vi "Write System Data.vi"(8 "Error In":errorcluster, 9 "AFV-P System Data":T1 {"Freq Lo Limit" format="%#.1f Hz"; "Freq Hi Limit" format="%#.1f Hz"; "Volt Lo Limit" format="%.1f V"; "Volt Hi Limit" format="%.1f V"; "DC Volt Lo Limit" format="%.1f V"; "DC Volt Hi Limit" format="%.1f V"}, 10 "Modbus ID":string, 11 "VISA resource name":refnum<visa-resource-name>) -> (0 "Error Out":errorcluster, 3 "VISA resource name out":refnum<visa-resource-name>)   [LabVIEW 2013]
panel:
  # "."
  # "."
  # "."
  # "."
  # "."
  # "."
  # "."
  # "."
  # "."
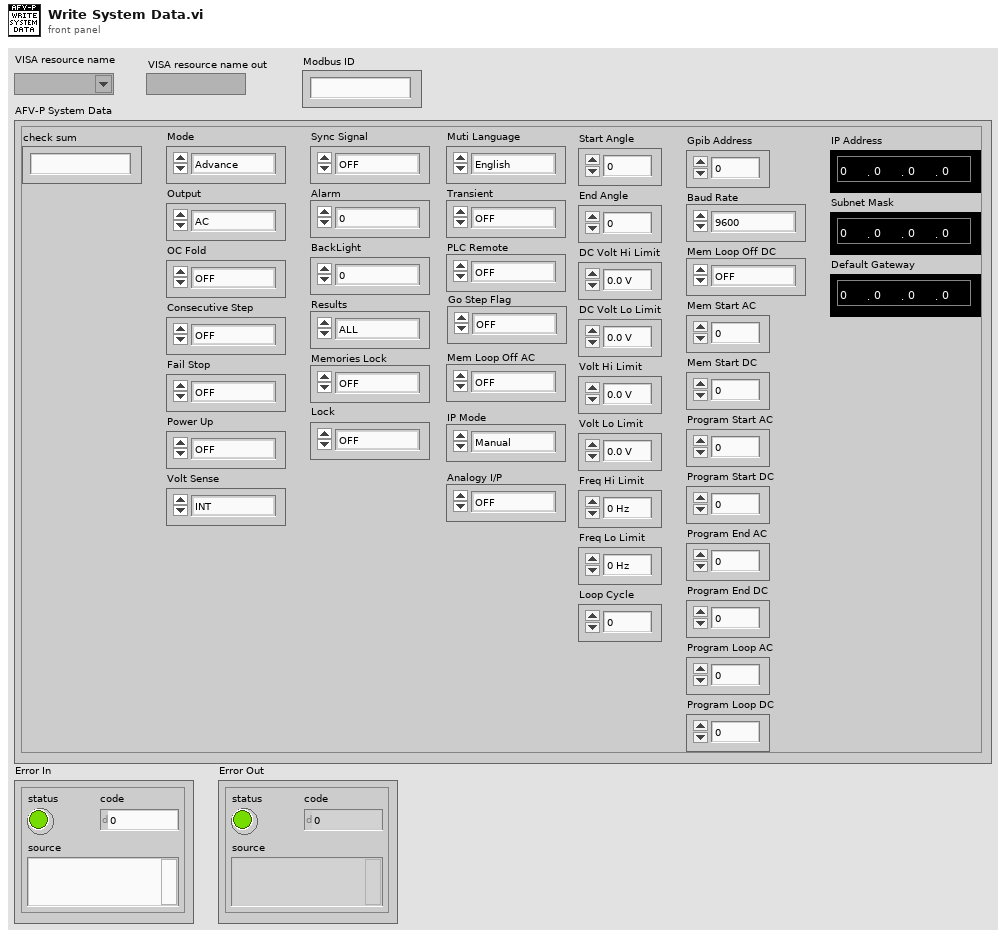
[diagram p1: front panel]
types:
  T1 = cluster{"check sum":string, "Mode":enum16{"Advance", "Basic"}, "Output":enum16{"AC", "DC"}, "OC Fold":enum16{"OFF", "ON"}, "Consecutive Step":enum16{"OFF", "ON"}, "Fail Stop":enum16{"OFF", "ON"}, "Power Up":enum16{"OFF", "ON", "LAST"}, "Volt Sense":enum16{"INT", "EXT"}, "Sync Signal":enum16{"OFF", "ON", "EVENT"}, "Alarm":enum16{"0", "1", "2", "3", "4", "5", "6", "7", "8", "9"}, "BackLight":enum16{"0", "1", "2", "3", "4", "5", "6", "7", "8", "9"}, "Results":enum16{"ALL", "P/F", "LAST"}, "Memories Lock":enum16{"OFF", "ON"}, "Lock":enum16{"OFF", "ON"}, "Muti Language":enum16{"English", "繁體中文", "簡體中文", "日文"}, "Transient":enum16{"OFF", "ON"}, "PLC Remote":enum16{"OFF", "ON"}, "Go Step Flag":enum16{"OFF", "ON"}, "Mem Loop Off AC":enum16{"OFF", "ON"}, "IP Mode":enum16{"Manual", "Auto"}, "Analogy I/P":enum16{"OFF", "ON"}, "Start Angle":u16, "End Angle":u16, "DC Volt Hi Limit":dbl, "DC Volt Lo Limit":dbl, "Volt Hi Limit":dbl, "Volt Lo Limit":dbl, "Freq Hi Limit":dbl, "Freq Lo Limit":dbl, "Loop Cycle":u16, "Gpib Address":u8, "Baud Rate":enum16{"9600", "19200", "38400", "57600", "115200"}, "Mem Loop Off DC":enum16{"OFF", "ON"}, "Mem Start AC":u8, "Mem Start DC":u8, "Program Start AC":u16, "Program Start DC":u16, "Program End AC":u16, "Program End DC":u16, "Program Loop AC":u16, "Program Loop DC":u16, "IP Address":cluster{"IP 0":u8, "IP 1":u8, "IP 2":u8, "IP 3":u8}, "Subnet Mask":cluster{"IP 0":u8, "IP 1":u8, "IP 2":u8, "IP 3":u8}, "Default Gateway":cluster{"IP 0":u8, "IP 1":u8, "IP 2":u8, "IP 3":u8}}
  T2 = cluster{"ID":string, "Function Code":string, "Length (High)":string, "Length (Low)":string, "Start Address (High)":string, "Start Address (Middle High)":string, "Start Address (Middle Low)":string, "Start Address (Low)":string, "Data":string}
  T3 = enum16{"0", "1", "2", "3", "4", "5", "6", "7", "8", "9"}
  T4 = enum16{"9600", "19200", "38400", "57600", "115200"}
  T5 = cluster{"Length (High)":string, "Length (Low)":string, "Start Address (High)":string, "Start Address (Middle High)":string, "Start Address (Middle Low)":string, "Start Address (Low)":string}
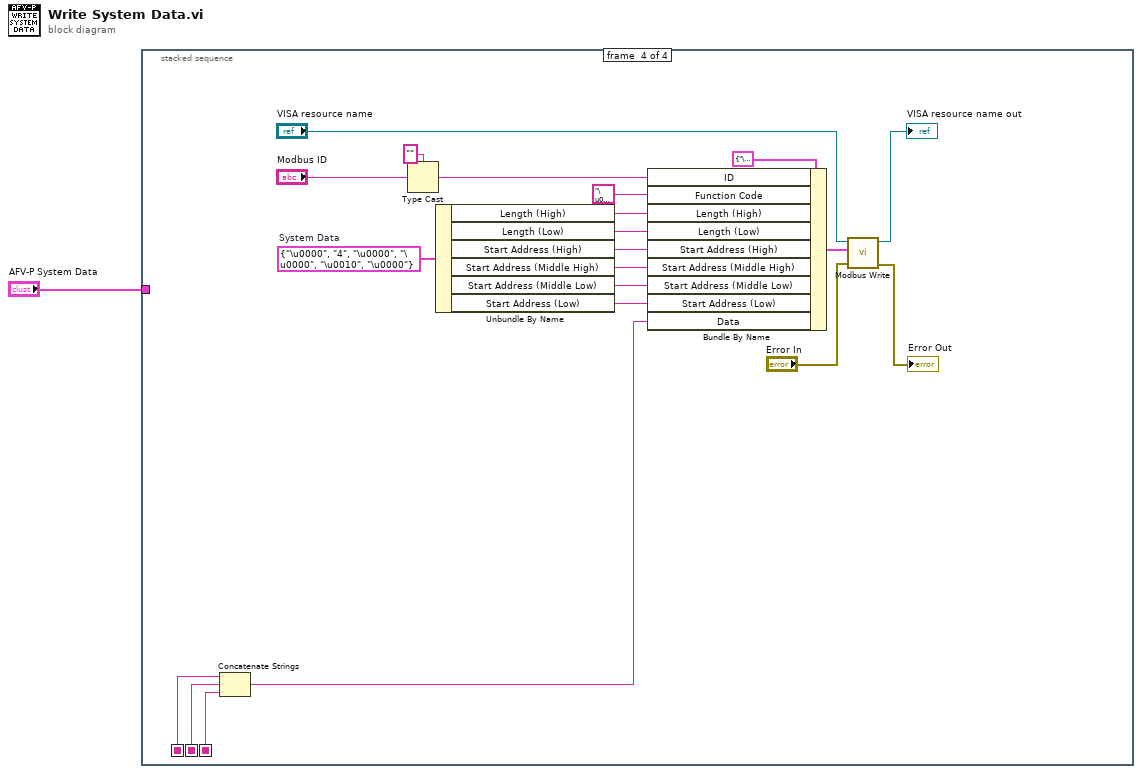
[diagram p0: block diagram]
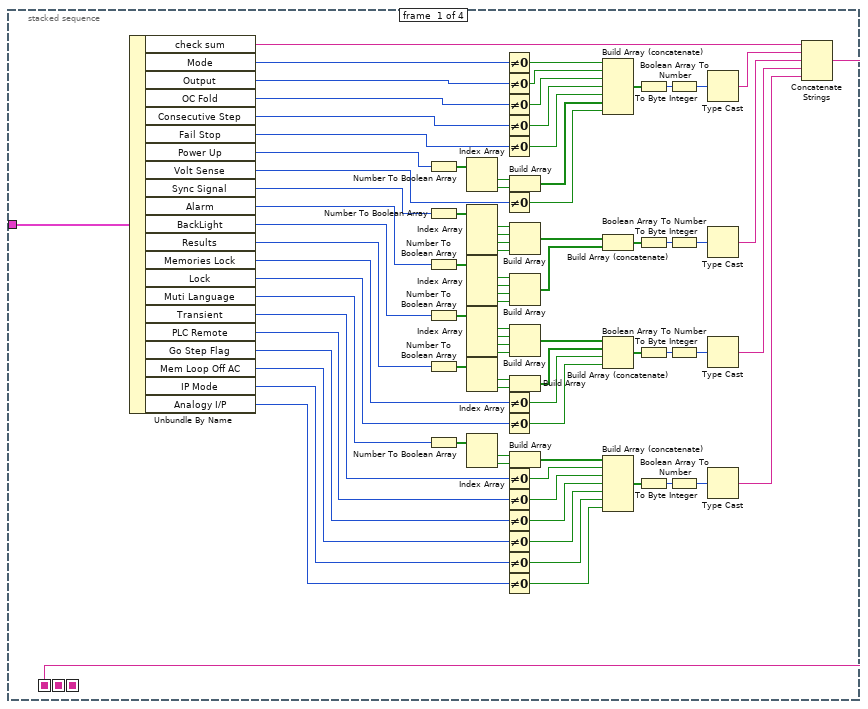
[diagram p2: hidden frame]
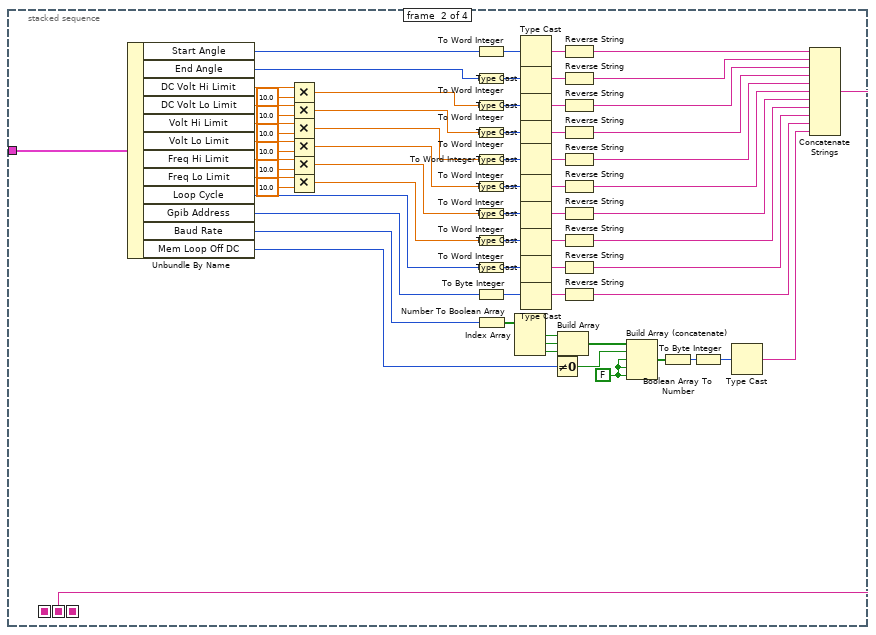
[diagram p3: hidden frame]
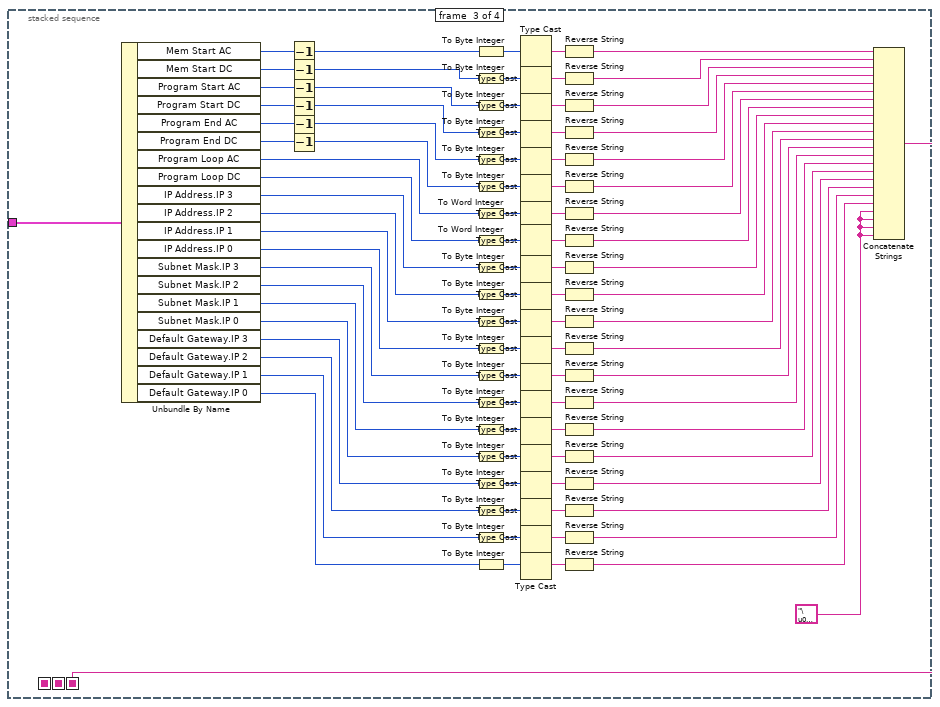
[diagram p4: hidden frame]
diagram:
  n1 = stacked-sequence {
    seq-local: [w11 _ _ _] -> [_ _ _ w261]
    seq-local: [_ w151 _ _] -> [_ _ _ w260]
    seq-local: [_ _ w217 _] -> [_ _ _ w259]
    tunnel: "AFV-P System Data" -> [w2 w85 w152 _]
    frame #0 {
      n2 = Unbundle By Name(w2) -> ("check sum"=w84:string, "Mode"=w83:enum16{"Advance", "Basic"}, "Output"=w82:enum16{"AC", "DC"}, "OC Fold"=w81:enum16{"OFF", "ON"}, "Consecutive Step"=w80:enum16{"OFF", "ON"}, "Fail Stop"=w79:enum16{"OFF", "ON"}, "Power Up"=w75:enum16{"OFF", "ON", "LAST"}, "Volt Sense"=w65:enum16{"INT", "EXT"}, "Sync Signal"=w59:enum16{"OFF", "ON", "EVENT"}, "Alarm"=w51:T3, "BackLight"=w39:T3, "Results"=w35:enum16{"ALL", "P/F", "LAST"}, "Memories Lock"=w34:enum16{"OFF", "ON"}, "Lock"=w33:enum16{"OFF", "ON"}, "Muti Language"=w21:enum16{"English", "繁體中文", "簡體中文", "日文"}, "Transient"=w20:enum16{"OFF", "ON"}, "PLC Remote"=w19:enum16{"OFF", "ON"}, "Go Step Flag"=w9:enum16{"OFF", "ON"}, "Mem Loop Off AC"=w8:enum16{"OFF", "ON"}, "IP Mode"=w7:enum16{"Manual", "Auto"}, "Analogy I/P"=w6:enum16{"OFF", "ON"})
      n3 = Number To Boolean Array(number=w75) -> (Boolean array=w78:bool[])
      n4 = Number To Boolean Array(number=w59) -> (Boolean array=w60:bool[])
      n5 = Number To Boolean Array(number=w51) -> (Boolean array=w54:bool[])
      n6 = Number To Boolean Array(number=w39) -> (Boolean array=w42:bool[])
      n7 = Number To Boolean Array(number=w35) -> (Boolean array=w36:bool[])
      n8 = Number To Boolean Array(number=w21) -> (Boolean array=w24:bool[])
      n9 = Index Array(array=w78) -> (element #1=w77:bool, element #2=w76:bool)  [unwired: 2 in]
      n10 = Index Array(array=w60) -> (element #1=w61:bool, element #2=w62:bool, element #3=w58:bool, element #4=w57:bool)  [unwired: 4 in]
      n11 = Index Array(array=w54) -> (element #1=w53:bool, element #2=w52:bool, element #3=w55:bool, element #4=w56:bool)  [unwired: 4 in]
      n12 = Index Array(array=w42) -> (element #1=w43:bool, element #2=w44:bool, element #3=w41:bool, element #4=w40:bool)  [unwired: 4 in]
      n13 = Index Array(array=w36) -> (element #1=w37:bool, element #2=w38:bool)  [unwired: 2 in]
      n14 = Index Array(array=w24) -> (element #1=w23:bool, element #2=w22:bool)  [unwired: 2 in]
      n15 = Not Equal To 0?(x=w83) -> (x != 0?=w71:bool)
      n16 = Not Equal To 0?(x=w82) -> (x != 0?=w70:bool)
      n17 = Not Equal To 0?(x=w81) -> (x != 0?=w69:bool)
      n18 = Not Equal To 0?(x=w80) -> (x != 0?=w68:bool)
      n19 = Not Equal To 0?(x=w79) -> (x != 0?=w67:bool)
      n20 = Not Equal To 0?(x=w65) -> (x != 0?=w64:bool)
      n21 = Not Equal To 0?(x=w34) -> (x != 0?=w30:bool)
      n22 = Not Equal To 0?(x=w33) -> (x != 0?=w29:bool)
      n23 = Not Equal To 0?(x=w20) -> (x != 0?=w14:bool)
      n24 = Not Equal To 0?(x=w19) -> (x != 0?=w13:bool)
      n25 = Not Equal To 0?(x=w9) -> (x != 0?=w10:bool)
      n26 = Not Equal To 0?(x=w8) -> (x != 0?=w5:bool)
      n27 = Not Equal To 0?(x=w7) -> (x != 0?=w4:bool)
      n28 = Not Equal To 0?(x=w6) -> (x != 0?=w3:bool)
      n29 = Build Array(w77, w76) -> (w66:bool[])
      n30 = Build Array(w61, w62, w58, w57) -> (w47:bool[])
      n31 = Build Array(w53, w52, w55, w56) -> (w46:bool[])
      n32 = Build Array(w43, w44, w41, w40) -> (w32:bool[])
      n33 = Build Array(w37, w38) -> (w31:bool[])
      n34 = Build Array(w23, w22) -> (w15:bool[])
      n35 = Build Array (concatenate)(w71, w70, w69, w68, w67, w66, w64) -> (w74:bool[])
      n36 = Build Array (concatenate)(w47, w46) -> (w48:bool[])
      n37 = Build Array (concatenate)(w32, w31, w30, w29) -> (w26:bool[])
      n38 = Build Array (concatenate)(w15, w14, w13, w10, w5, w4, w3) -> (w18:bool[])
      n39 = Boolean Array To Number(Boolean array=w74) -> (number=w73:u32)
      n40 = Boolean Array To Number(Boolean array=w48) -> (number=w49:u32)
      n41 = Boolean Array To Number(Boolean array=w26) -> (number=w28:u32)
      n42 = Boolean Array To Number(Boolean array=w18) -> (number=w16:u32)
      n43 = To Byte Integer(number=w73) -> (8bit integer=w72:i8)
      n44 = To Byte Integer(number=w49) -> (8bit integer=w50:i8)
      n45 = To Byte Integer(number=w28) -> (8bit integer=w27:i8)
      n46 = To Byte Integer(number=w16) -> (8bit integer=w17:i8)
      n47 = Type Cast(x=w72) -> (*(type *) &x=w63:string)  [unwired: 1 in]
      n48 = Type Cast(x=w50) -> (*(type *) &x=w45:string)  [unwired: 1 in]
      n49 = Type Cast(x=w27) -> (*(type *) &x=w25:string)  [unwired: 1 in]
      n50 = Type Cast(x=w17) -> (*(type *) &x=w12:string)  [unwired: 1 in]
      n51 = Concatenate Strings(w84, w63, w45, w25, w12) -> (w11:string)
    }
    frame #1 {
      w98 = FALSE
      n52 = Unbundle By Name(w85) -> ("Start Angle"=w148:u16, "End Angle"=w144:u16, "DC Volt Hi Limit"=w102:dbl, "DC Volt Lo Limit"=w100:dbl, "Volt Hi Limit"=w111:dbl, "Volt Lo Limit"=w119:dbl, "Freq Hi Limit"=w116:dbl, "Freq Lo Limit"=w114:dbl, "Loop Cycle"=w128:u16, "Gpib Address"=w123:u8, "Baud Rate"=w88:T4, "Mem Loop Off DC"=w87:enum16{"OFF", "ON"})
      n53 = Multiply(x=w102, y=10.0) -> (x*y=w101:dbl)
      n54 = Multiply(x=w100, y=10.0) -> (x*y=w99:dbl)
      n55 = Multiply(x=w111, y=10.0) -> (x*y=w121:dbl)
      n56 = Multiply(x=w119, y=10.0) -> (x*y=w118:dbl)
      n57 = Multiply(x=w116, y=10.0) -> (x*y=w115:dbl)
      n58 = Multiply(x=w114, y=10.0) -> (x*y=w112:dbl)
      n59 = To Word Integer(number=w148) -> (16bit integer=w149:i16)
      n60 = To Word Integer(number=w144) -> (16bit integer=w146:i16)
      n61 = To Word Integer(number=w101) -> (16bit integer=w108:i16)
      n62 = To Word Integer(number=w99) -> (16bit integer=w109:i16)
      n63 = To Word Integer(number=w121) -> (16bit integer=w141:i16)
      n64 = To Word Integer(number=w118) -> (16bit integer=w139:i16)
      n65 = To Word Integer(number=w115) -> (16bit integer=w135:i16)
      n66 = To Word Integer(number=w112) -> (16bit integer=w133:i16)
      n67 = To Word Integer(number=w128) -> (16bit integer=w129:i16)
      n68 = To Byte Integer(number=w123) -> (8bit integer=w126:i8)
      n69 = Number To Boolean Array(number=w88) -> (Boolean array=w95:bool[])
      n70 = Index Array(array=w95) -> (element #1=w96:bool, element #2=w97:bool, element #3=w94:bool)  [unwired: 3 in]
      n71 = Type Cast(x=w149) -> (*(type *) &x=w150:string)  [unwired: 1 in]
      n72 = Type Cast(x=w146) -> (*(type *) &x=w145:string)  [unwired: 1 in]
      n73 = Type Cast(x=w108) -> (*(type *) &x=w107:string)  [unwired: 1 in]
      n74 = Type Cast(x=w109) -> (*(type *) &x=w110:string)  [unwired: 1 in]
      n75 = Type Cast(x=w141) -> (*(type *) &x=w142:string)  [unwired: 1 in]
      n76 = Type Cast(x=w139) -> (*(type *) &x=w138:string)  [unwired: 1 in]
      n77 = Type Cast(x=w135) -> (*(type *) &x=w136:string)  [unwired: 1 in]
      n78 = Type Cast(x=w133) -> (*(type *) &x=w132:string)  [unwired: 1 in]
      n79 = Type Cast(x=w129) -> (*(type *) &x=w130:string)  [unwired: 1 in]
      n80 = Type Cast(x=w126) -> (*(type *) &x=w125:string)  [unwired: 1 in]
      n81 = Not Equal To 0?(x=w87) -> (x != 0?=w86:bool)
      n82 = Build Array(w96, w97, w94) -> (w93:bool[])
      n83 = Reverse String(1:w150) -> (0:w147:string)
      n84 = Reverse String(1:w145) -> (0:w143:string)
      n85 = Reverse String(1:w107) -> (0:w106:string)
      n86 = Reverse String(1:w110) -> (0:w105:string)
      n87 = Reverse String(1:w142) -> (0:w140:string)
      n88 = Reverse String(1:w138) -> (0:w137:string)
      n89 = Reverse String(1:w136) -> (0:w134:string)
      n90 = Reverse String(1:w132) -> (0:w131:string)
      n91 = Reverse String(1:w130) -> (0:w127:string)
      n92 = Reverse String(1:w125) -> (0:w124:string)
      n93 = Build Array (concatenate)(w93, w86, w98, w98, w98) -> (w90:bool[])
      n94 = Boolean Array To Number(Boolean array=w90) -> (number=w92:u32)
      n95 = To Byte Integer(number=w92) -> (8bit integer=w91:i8)
      n96 = Type Cast(x=w91) -> (*(type *) &x=w89:string)  [unwired: 1 in]
      n97 = Concatenate Strings(w147, w143, w106, w105, w140, w137, w134, w131, w127, w124, w89) -> (w151:string)
    }
    frame #2 {
      w176 = "\u0000" ("string")
      n98 = Unbundle By Name(w152) -> ("Mem Start AC"=w238:u8, "Mem Start DC"=w232:u8, "Program Start AC"=w231:u16, "Program Start DC"=w159:u16, "Program End AC"=w158:u16, "Program End DC"=w157:u16, "Program Loop AC"=w156:u16, "Program Loop DC"=w160:u16, "IP Address.IP 3"=w216:u8, "IP Address.IP 2"=w215:u8, "IP Address.IP 1"=w214:u8, "IP Address.IP 0"=w194:u8, "Subnet Mask.IP 3"=w193:u8, "Subnet Mask.IP 2"=w192:u8, "Subnet Mask.IP 1"=w191:u8, "Subnet Mask.IP 0"=w190:u8, "Default Gateway.IP 3"=w189:u8, "Default Gateway.IP 2"=w188:u8, "Default Gateway.IP 1"=w187:u8, "Default Gateway.IP 0"=w186:u8)
      n99 = Decrement(x=w238) -> (x-1=w167:u8)
      n100 = Decrement(x=w232) -> (x-1=w219:u8)
      n101 = Decrement(x=w231) -> (x-1=w218:u16)
      n102 = Decrement(x=w159) -> (x-1=w155:u16)
      n103 = Decrement(x=w158) -> (x-1=w154:u16)
      n104 = Decrement(x=w157) -> (x-1=w153:u16)
      n105 = To Byte Integer(number=w167) -> (8bit integer=w240:i8)
      n106 = To Byte Integer(number=w219) -> (8bit integer=w233:i8)
      n107 = To Byte Integer(number=w218) -> (8bit integer=w236:i8)
      n108 = To Byte Integer(number=w155) -> (8bit integer=w170:i8)
      n109 = To Byte Integer(number=w154) -> (8bit integer=w175:i8)
      n110 = To Byte Integer(number=w153) -> (8bit integer=w172:i8)
      n111 = To Word Integer(number=w156) -> (16bit integer=w168:i16)
      n112 = To Word Integer(number=w160) -> (16bit integer=w230:i16)
      n113 = To Byte Integer(number=w216) -> (8bit integer=w227:i8)
      n114 = To Byte Integer(number=w215) -> (8bit integer=w224:i8)
      n115 = To Byte Integer(number=w214) -> (8bit integer=w213:i8)
      n116 = To Byte Integer(number=w194) -> (8bit integer=w208:i8)
      n117 = To Byte Integer(number=w193) -> (8bit integer=w211:i8)
      n118 = To Byte Integer(number=w192) -> (8bit integer=w212:i8)
      n119 = To Byte Integer(number=w191) -> (8bit integer=w196:i8)
      n120 = To Byte Integer(number=w190) -> (8bit integer=w199:i8)
      n121 = To Byte Integer(number=w189) -> (8bit integer=w200:i8)
      n122 = To Byte Integer(number=w188) -> (8bit integer=w205:i8)
      n123 = To Byte Integer(number=w187) -> (8bit integer=w202:i8)
      n124 = To Byte Integer(number=w186) -> (8bit integer=w201:i8)
      n125 = Type Cast(x=w240) -> (*(type *) &x=w239:string)  [unwired: 1 in]
      n126 = Type Cast(x=w233) -> (*(type *) &x=w234:string)  [unwired: 1 in]
      n127 = Type Cast(x=w236) -> (*(type *) &x=w235:string)  [unwired: 1 in]
      n128 = Type Cast(x=w170) -> (*(type *) &x=w171:string)  [unwired: 1 in]
      n129 = Type Cast(x=w175) -> (*(type *) &x=w174:string)  [unwired: 1 in]
      n130 = Type Cast(x=w172) -> (*(type *) &x=w173:string)  [unwired: 1 in]
      n131 = Type Cast(x=w168) -> (*(type *) &x=w169:string)  [unwired: 1 in]
      n132 = Type Cast(x=w230) -> (*(type *) &x=w229:string)  [unwired: 1 in]
      n133 = Type Cast(x=w227) -> (*(type *) &x=w226:string)  [unwired: 1 in]
      n134 = Type Cast(x=w224) -> (*(type *) &x=w225:string)  [unwired: 1 in]
      n135 = Type Cast(x=w213) -> (*(type *) &x=w228:string)  [unwired: 1 in]
      n136 = Type Cast(x=w208) -> (*(type *) &x=w209:string)  [unwired: 1 in]
      n137 = Type Cast(x=w211) -> (*(type *) &x=w210:string)  [unwired: 1 in]
      n138 = Type Cast(x=w212) -> (*(type *) &x=w207:string)  [unwired: 1 in]
      n139 = Type Cast(x=w196) -> (*(type *) &x=w197:string)  [unwired: 1 in]
      n140 = Type Cast(x=w199) -> (*(type *) &x=w198:string)  [unwired: 1 in]
      n141 = Type Cast(x=w200) -> (*(type *) &x=w195:string)  [unwired: 1 in]
      n142 = Type Cast(x=w205) -> (*(type *) &x=w204:string)  [unwired: 1 in]
      n143 = Type Cast(x=w202) -> (*(type *) &x=w203:string)  [unwired: 1 in]
      n144 = Type Cast(x=w201) -> (*(type *) &x=w206:string)  [unwired: 1 in]
      n145 = Reverse String(1:w239) -> (0:w237:string)
      n146 = Reverse String(1:w234) -> (0:w166:string)
      n147 = Reverse String(1:w235) -> (0:w165:string)
      n148 = Reverse String(1:w171) -> (0:w164:string)
      n149 = Reverse String(1:w174) -> (0:w163:string)
      n150 = Reverse String(1:w173) -> (0:w162:string)
      n151 = Reverse String(1:w169) -> (0:w161:string)
      n152 = Reverse String(1:w229) -> (0:w223:string)
      n153 = Reverse String(1:w226) -> (0:w222:string)
      n154 = Reverse String(1:w225) -> (0:w221:string)
      n155 = Reverse String(1:w228) -> (0:w220:string)
      n156 = Reverse String(1:w209) -> (0:w185:string)
      n157 = Reverse String(1:w210) -> (0:w184:string)
      n158 = Reverse String(1:w207) -> (0:w183:string)
      n159 = Reverse String(1:w197) -> (0:w182:string)
      n160 = Reverse String(1:w198) -> (0:w181:string)
      n161 = Reverse String(1:w195) -> (0:w180:string)
      n162 = Reverse String(1:w204) -> (0:w179:string)
      n163 = Reverse String(1:w203) -> (0:w178:string)
      n164 = Reverse String(1:w206) -> (0:w177:string)
      n165 = Concatenate Strings(w237, w166, w165, w164, w163, w162, w161, w223, w222, w221, w220, w185, w184, w183, w182, w181, w180, w179, w178, w177, w176, w176, w176, w176) -> (w217:string)
    }
    frame #3 {
      w258 = T5 {"Length (High)"="\u0000", "Length (Low)"="4", "Start Address (High)"="\u0000", "Start Address (Middle High)"="\u0000", "Start Address (Middle Low)"="\u0010", "Start Address (Low)"="\u0000"}  # System Data
      n166 = Concatenate Strings(w261, w260, w259) -> (w241:string)
      n167 = Type Cast(type="" ("Binary Data (Hex) 3"), x="Modbus ID") -> (*(type *) &x=w257:string)
      n168 = Unbundle By Name(w258) -> ("Length (High)"=w250:string, "Length (Low)"=w249:string, "Start Address (High)"=w248:string, "Start Address (Middle High)"=w247:string, "Start Address (Middle Low)"=w246:string, "Start Address (Low)"=w245:string)
      n169 = Bundle By Name(cluster=T2 {"ID"="\u0000", "Function Code"="\u0000", "Length (High)"="\u0000", "Length (Low)"="\u0000", "Start Address (High)"="\u0000", "Start Address (Middle High)"="\u0000", "Start Address (Middle Low)"="\u0000", "Start Address (Low)"="\u0000", "Data"=""} ("Write Buffer"), "ID"=w257, "Function Code"="\u0010", "Length (High)"=w250, "Length (Low)"=w249, "Start Address (High)"=w248, "Start Address (Middle High)"=w247, "Start Address (Middle Low)"=w246, "Start Address (Low)"=w245, "Data"=w241) -> (w252:T2)
      n170 = call "Modbus Write.vi"("Error In"="Error In", "Write Buffer"=w252, "VISA resource name"="VISA resource name") -> ("Error Out"=→"Error Out":errorcluster, "VISA resource name out"=→"VISA resource name out":refnum<visa-resource-name>)  [unwired: 7 in]
    }
  }
